vi "Climb Mode Select.vi"(10 "D-Pad":T2, 11 "Manipulator Axes":T1) -> (0 "Winch":dbl, 1 "Climb?":bool, 2 "Fire?":bool, 3 "Extend?":bool)   [LabVIEW 2015]
uses:
  Common Code/Gamepads/D-Pad.ctl
  Common Code/Gamepads/Axes Cluster.ctl
  Common Code/Change Detect.vi
  Common Code/Change Detect Boolean.vi
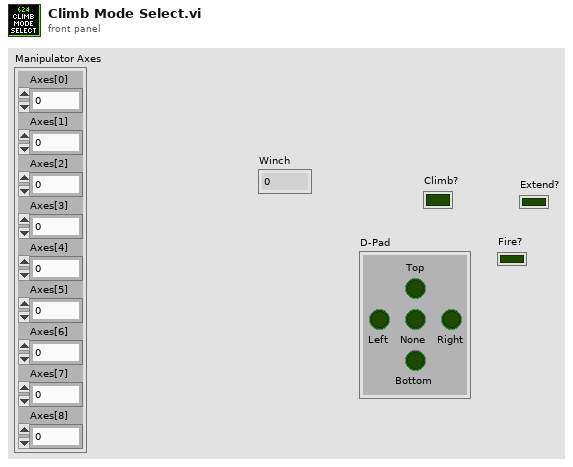
[diagram p1: front panel]
types:
  T1 = typedef "Axes Cluster.ctl" = cluster{"Axes[0]":dbl, "Axes[1]":dbl, "Axes[2]":dbl, "Axes[3]":dbl, "Axes[4]":dbl, "Axes[5]":dbl, "Axes[6]":dbl, "Axes[7]":dbl, "Axes[8]":dbl}
  T2 = typedef "D-Pad.ctl" = cluster{"Top":bool, "Bottom":bool, "None":bool, "Right":bool, "Left":bool}
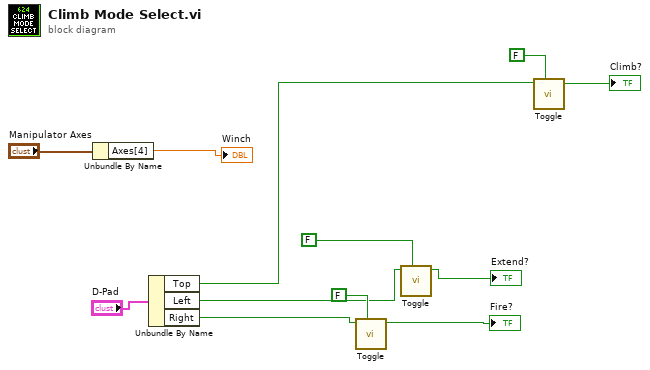
[diagram p0: block diagram]
diagram:
  n1 = Unbundle By Name("Manipulator Axes") -> ("Axes[4]"=→"Winch":dbl)
  n2 = Unbundle By Name("D-Pad") -> ("Top"=w3:bool, "Left"=w6:bool, "Right"=w4:bool)
  n3 = call "Toggle.vi"("Initial Value"=FALSE, "In"=w4) -> ("Toggled"=→"Fire?":bool)  [unwired: 9 in]
  n4 = call "Toggle.vi"("Initial Value"=FALSE, "In"=w6) -> ("Toggled"=→"Extend?":bool)  [unwired: 9 in]
  n5 = call "Toggle.vi"("Initial Value"=FALSE, "In"=w3) -> ("Toggled"=→"Climb?":bool)  [unwired: 9 in]
